vi "TracePoint_UnhandledMessage.vi"(8 "error in (no error)":errorcluster, 10 "message":string, 11 "Qbus in":refnum<class "Qbus.lvclass">) -> (0 "error out":errorcluster)   [LabVIEW 2017, in "IrDataEventCreator.lvlib"]
uses:
  <vilib>/addons/InsightCM/Devices/Shared/Ir/IrDataEventCreator/IrDataEventCreator.lvlib
  <vilib>/addons/Qbus/Qbus.lvclass
  <vilib>/addons/TraceLogger/TraceLogger.lvlib
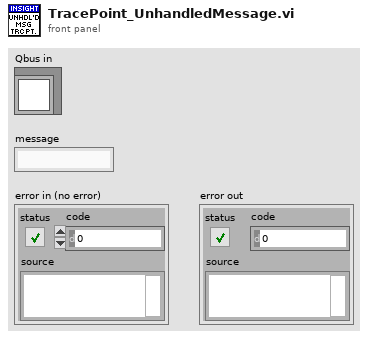
[diagram p1: front panel]
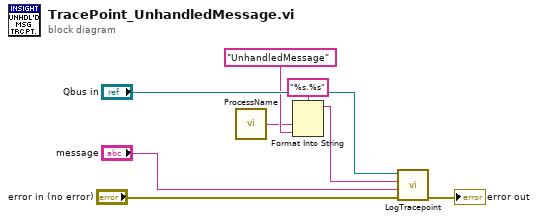
[diagram p0: block diagram]
diagram:
  n1 = call <vilib>:"ProcessName.vi"() -> ("process name"=w3:string)  [unwired: 5 in]
  n2 = Format Into String(format string="%s.%s", w3, "UnhandledMessage" ("tracepoint")) -> (resulting string=w1:string)  [unwired: 2 in, 1 out]
  n3 = call <vilib>:"LogTracepoint.vi"("error in (no error)"="error in (no error)", "log string"="message", "tracepoint"=w1, "qbus in"="Qbus in") -> ("error out"=→"error out":errorcluster)  [unwired: 6 in, 1 out]
